vi "Select System.vi"(8 "Error In":errorcluster, 9 "LowerRackSerialNumber":string="Please Place in Rack ", 10 "UpperRackSerialNumber":string="Please Place in Rack ", 11 "connection information":path) -> (0 "Error Out":errorcluster, 1 "NewLowerRackNumber":string, 2 "NewUpperRackNumber":string, 4 "NewSystem":string, 6 "Move?":bool)   [LabVIEW 2024]
uses:
  <vilib>/addons/database/Connection.llb/DB Tools Open Connec (Path).vi
  <vilib>/addons/database/_DB Variant To Data/Database Variant To Data.xnode
  <vilib>/addons/database/NI_Database_API.lvlib
panel:
  in  "Ok":bool
  in  "System Number":string(combo)="1000"
  # "Please Select New System\nfor Boards"
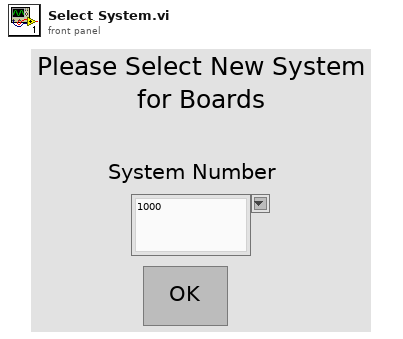
[diagram p1: front panel]
types:
  T1 = typedef "NI_Database_API.lvlib/Conn ObjectReference.ctl" = refnum<k1>
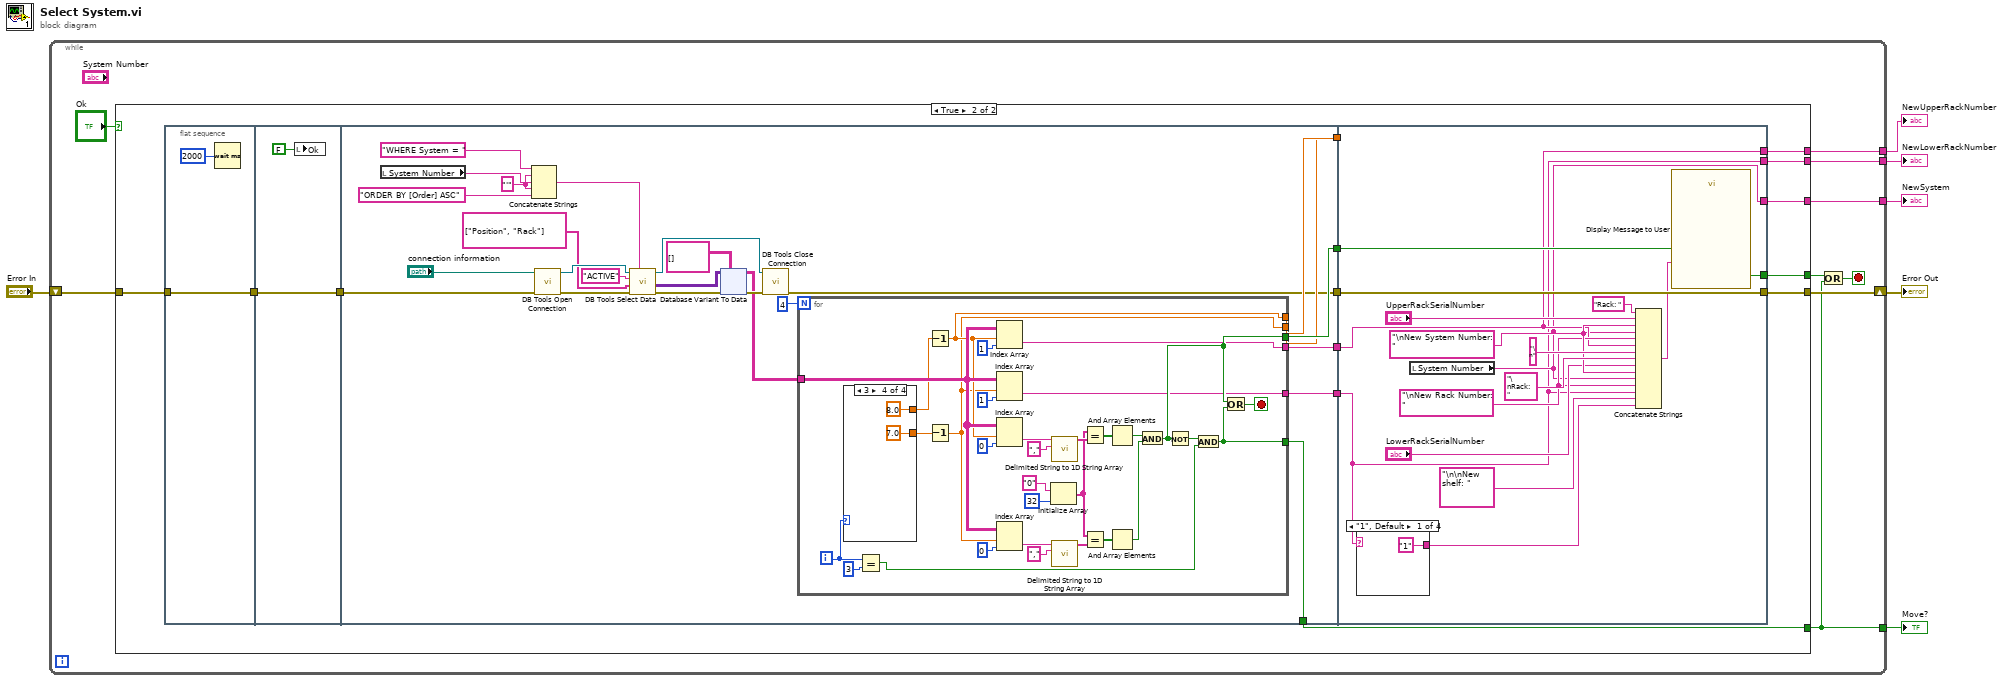
[diagram p0: block diagram]
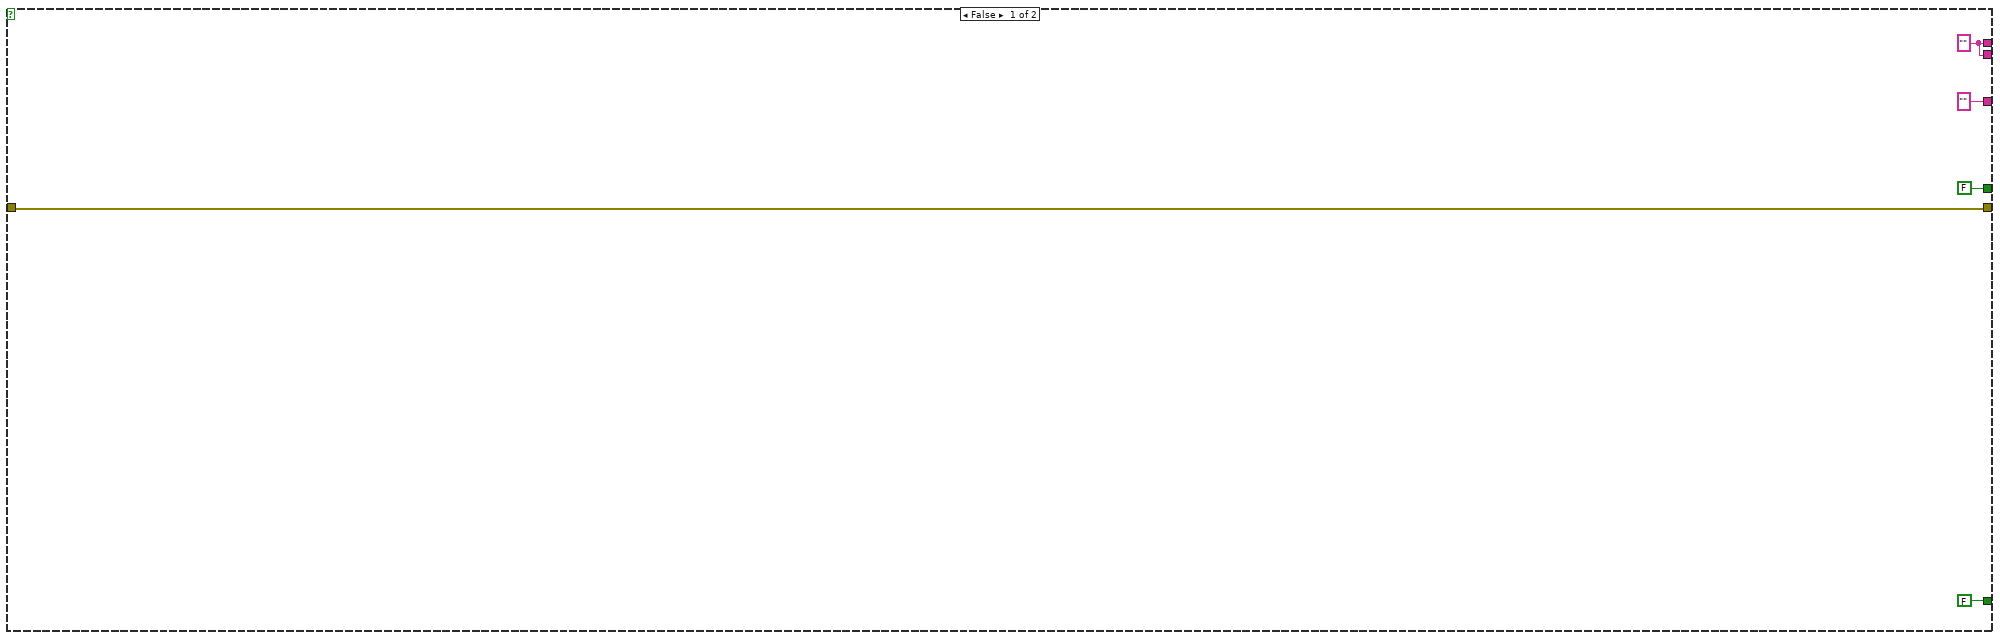
[diagram p2: hidden frame]
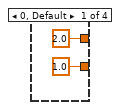
[diagram p3: hidden frame]
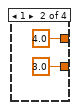
[diagram p4: hidden frame]
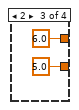
[diagram p5: hidden frame]
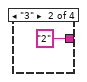
[diagram p6: hidden frame]
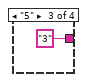
[diagram p7: hidden frame]
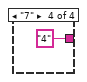
[diagram p8: hidden frame]
diagram:
  n1 = while {
    shift-right: [w13] -> w5
    shift-left: "Error In" -> [w14]
    tunnel: [w11] -> w4
    tunnel: [w9] -> w3
    tunnel: [w8] -> w2
    tunnel: [w7] -> w1
    stop <- w10 stop-if-true
    n2 = case shown="True" "Ok" {
      tunnel: w14 -> [w20 w35]
      tunnel: [w20 w34] -> w13
      tunnel: [FALSE ("Yes") w32] -> w12
      tunnel: [FALSE w31] -> w8
      tunnel: [w17 w24] -> w11
      tunnel: [w17 w25] -> w9
      tunnel: ["" w23] -> w7
      frame False {
        w17 = "" ("String")
      }
      frame True {
        n3 = flat-sequence {
          tunnel: w35 -> [w37]
          tunnel: [w37] -> w21
          tunnel: [w39] -> w22
          tunnel: w21 -> [w39]
          tunnel: [w43] -> w33
          tunnel: [w59] -> w31
          tunnel: [w64] -> w30
          tunnel: [w63] -> w29
          tunnel: [w62] -> w28
          tunnel: [w61] -> w27
          tunnel: [w60] -> w26
          tunnel: w22 -> [w44]
          tunnel: [w163] -> w34
          tunnel: w33 -> [w163]
          tunnel: [w162] -> w32
          tunnel: w30 -> [w160]
          tunnel: w29 -> [_]
          tunnel: w28 -> [_]
          tunnel: w27 -> [w152]
          tunnel: w26 -> [w149]
          tunnel: [w149] -> w25
          tunnel: [w152] -> w24
          tunnel: [w151] -> w23
          frame #0 {
            n4 = Wait (ms)(milliseconds to wait=u32 2000) -> ()  [unwired: 1 out]
          }
          frame #1 {
            n5 = local write "Ok"(FALSE ("Ok")) -> ()
          }
          frame #2 {
            w56 = "'" ("string")
            n6 = local read "System Number"() -> (w55:string)
            n7 = Concatenate Strings("WHERE System = " ("SQL Query"), w56, w55, w56, "ORDER BY [Order] ASC" ("string")) -> (w45:string)
            n8 = call-poly <vilib>:"DB Tools Open Connection.vi"("error in (no error)"=w44, "connection information"="connection information") -> ("error out"=w51:errorcluster, "connection reference"=w53:T1)  [unwired: 6 in]
            n9 = call <vilib>:"DB Tools Select Data.vi"("condition"=w45, "error in (no error)"=w51, "columns"=string[] ["Position", "Rack"], "table"="ACTIVE", "connection reference"=w53) -> ("error out"=w50:errorcluster, "data"=w48:variant[][], "connection reference out"=w52:T1)  [unwired: 1 in]
            n10 = xnode "Database Variant To Data"("database variant"=w48, "error in (no error)"=w50, "type"=string[][] [] ("delimiter")) -> ("data"=w46:string[][], "error out"=w49:errorcluster)
            n11 = call <vilib>:"DB Tools Close Connection.vi"("error in (no error)"=w49, "connection reference"=w52) -> ("error out"=w43:errorcluster)  [unwired: 5 in]
            n12 = for {
              N: 4 -> [_]
              tunnel: w46 -> [w126]
              tunnel: [w110] -> w61
              tunnel: [w118] -> w64
              tunnel: [w109] -> w60
              tunnel: [w113] -> w63
              tunnel: [w111] -> w62
              tunnel: [w116] -> w59
              i -> [w115]
              stop <- w130 stop-if-true
              n13 = case shown="3" w115 {
                tunnel: [1.0 3.0 5.0 7.0] -> w112
                tunnel: [2.0 4.0 6.0 8.0] -> w114
                frame 0, Default {
                }
                frame 1 {
                }
                frame 2 {
                }
                frame 3 {
                }
              }
              n14 = Equal?(x=w115, y=3) -> (x = y?=w117:bool)
              n15 = Decrement(x=w114) -> (x-1=w113:dbl)
              n16 = Decrement(x=w112) -> (x-1=w111:dbl)
              n17 = Index Array(array=w126, index (row)=w113, index (col)=1) -> (element=w110:string)
              n18 = Index Array(array=w126, index (row)=w111, index (col)=1) -> (element=w109:string)
              n19 = Index Array(array=w126, index (row)=w113, index (col)=0 ("disabled index (col)")) -> (element=w122:string)
              n20 = Index Array(array=w126, index (row)=w111, index (col)=0 ("disabled index (col)")) -> (element=w138:string)
              n21 = Initialize Array("0", 32 ("dimension size")) -> (w121:string[])
              n22 = call <vilib>:"Delimited String to 1D String Array.vi"("delimiter"=",", "delimited string"=w122) -> ("string array"=w124:string[])  [unwired: 9 in]
              n23 = call <vilib>:"Delimited String to 1D String Array.vi"("delimiter"=",", "delimited string"=w138) -> ("string array"=w134:string[])  [unwired: 9 in]
              n24 = Equal?(x=w121, y=w124) -> (x = y?=w123:bool[])
              n25 = Equal?(x=w121, y=w134) -> (x = y?=w132:bool[])
              n26 = And Array Elements(Boolean array=w123) -> (logical AND=w120:bool)
              n27 = And Array Elements(Boolean array=w132) -> (logical AND=w119:bool)
              n28 = And(x=w120, y=w119) -> (x .and. y?=w118:bool)
              n29 = Not(x=w118) -> (.not. x?=w129:bool)
              n30 = And(x=w129, y=w117) -> (x .and. y?=w116:bool)
              n31 = Or(x=w118, y=w116) -> (x .or. y?=w130:bool)
            }
          }
          frame #3 {
            w155 = "\nNew System Number: " ("string")
            w153 = "\nNew Rack Number: " ("string")
            n32 = case shown="\"1\", Default" w149 {
              tunnel: ["1" ("string") "2" ("string") "3" ("string") "4" ("string")] -> w148
              frame "1", Default {
              }
              frame "3" {
              }
              frame "5" {
              }
              frame "7" {
              }
            }
            n33 = local read "System Number"() -> (w151:string)
            n34 = Concatenate Strings("Rack: " ("Message"), "UpperRackSerialNumber", w155, w151, w153, w152, "\n" ("string"), "\nRack: " ("Message"), "LowerRackSerialNumber", w155, w151, w153, w149, "\n\nNew shelf: " ("string"), w148) -> (w161:string)
            n35 = call "Display Message to User"("Enable"=w160, "Message"=w161) -> ("Ok"=w162:bool)  [unwired: 8 in, 1 out]
          }
        }
      }
    }
    n36 = Or(x=w12, y=w8) -> (x .or. y?=w10:bool)
  }
  "Error Out" <- w5
  "NewUpperRackNumber" <- w4
  "Move?" <- w2
  "NewSystem" <- w1
  "NewLowerRackNumber" <- w3
